vi "Rectangle Comparison.vi"(9 "Second":dbl[](array[numeric]), 11 "First":dbl[](array[numeric])) -> (0 "Rect":T1, 3 "Scores":T2)   [LabVIEW 2017]
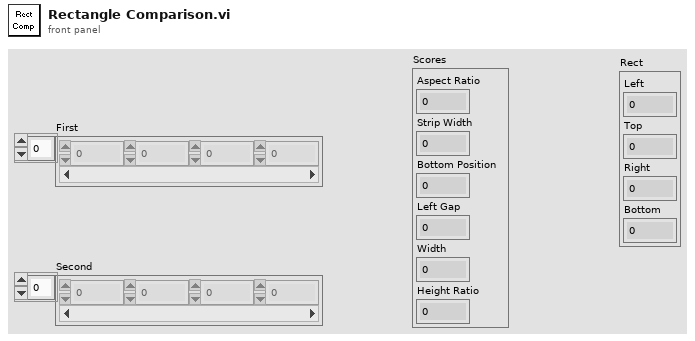
[diagram p1: front panel]
types:
  T1 = cluster{"Left":dbl, "Top":dbl, "Right":dbl, "Bottom":dbl}
  T2 = cluster{"Aspect Ratio":dbl, "Strip Width":dbl, "Bottom Position":dbl, "Left Gap":dbl, "Width":dbl, "Height Ratio":dbl}
  T3 = cluster{"[0]":dbl, "[1]":dbl, "[2]":dbl, "[3]":dbl}
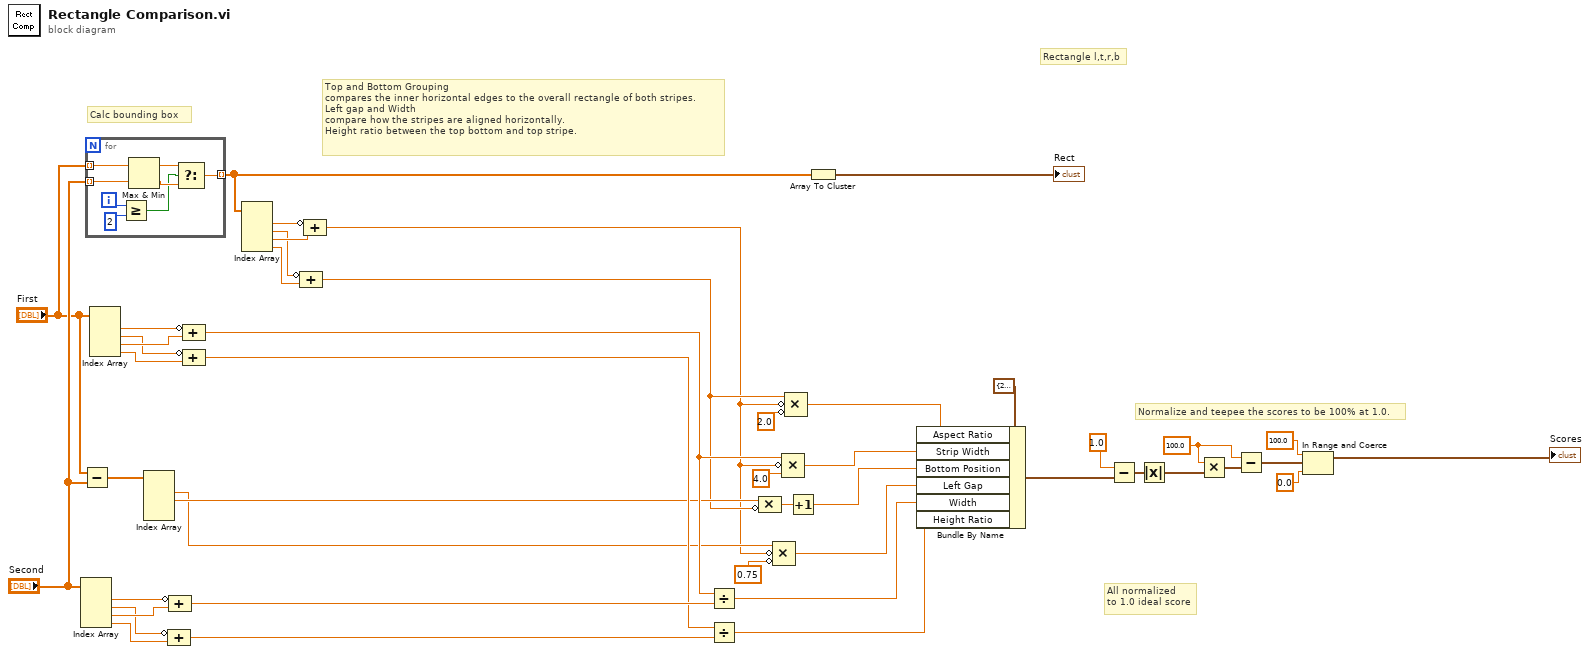
[diagram p0: block diagram]
diagram:
  w33 = 100.0 ("x/y")
  # "All normalized\nto 1.0 ideal score"
  # "Normalize and teepee the scores to be 100% at 1.0."
  # "Top and Bottom Grouping\ncompares the inner horizontal edges to the overall rectangle of both stripes.\nLeft gap and Width\ncompare how the stripes are aligned horizontally.\nHeight ratio between the top bottom and top stripe."
  # "Calc bounding box"
  # "Rectangle l,t,r,b"
  n1 = Index Array(array="Second") -> (element #1=w43:dbl, element #2=w24:dbl, element #3=w46:dbl, element #4=w8:dbl)  [unwired: 4 in]
  n2 = Subtract(x="First", y="Second") -> (x-y=w15:dbl[])
  n3 = for {
    tunnel: "First" -> [w54] mode=indexing
    tunnel: "Second" -> [w53] mode=indexing
    tunnel: [w47] -> w18 mode=indexing
    i -> [w51]
    n4 = Greater Or Equal?(x=w51, y=2) -> (x >= y?=w48:bool)
    n5 = Max & Min(x=w54, y=w53) -> (max(x,y)=w50:dbl, min(x,y)=w49:dbl)
    n6 = Select(t=w50, s=w48, f=w49) -> (s? t:f=w47:dbl)
  }
  n7 = Index Array(array="First") -> (element #1=w38:dbl, element #2=w23:dbl, element #3=w37:dbl, element #4=w39:dbl)  [unwired: 4 in]
  n8 = Index Array(array=w15) -> (element #1=w13:dbl, element #2=w14:dbl)  [unwired: 4 in, 2 out]
  n9 = Compound Arithmetic op=ADD(invert w24, w8) -> (w44:dbl)
  n10 = Compound Arithmetic op=ADD(invert w43, w46) -> (w45:dbl)
  n11 = Compound Arithmetic op=ADD(invert w38, w37) -> (w21:dbl)
  n12 = Compound Arithmetic op=ADD(invert w23, w39) -> (w25:dbl)
  n13 = Index Array(array=w18) -> (element #1=w10:dbl, element #2=w7:dbl, element #3=w9:dbl, element #4=w6:dbl)  [unwired: 4 in]
  n14 = Compound Arithmetic op=ADD(invert w7, w6) -> (w5:dbl)
  n15 = Compound Arithmetic op=ADD(invert w10, w9) -> (w4:dbl)
  n16 = Divide(x=w21, y=w45) -> (x/y=w41:dbl)
  n17 = Divide(x=w25, y=w44) -> (x/y=w40:dbl)
  n18 = Compound Arithmetic op=MULTIPLY(w14, invert w5) -> (w20:dbl)
  n19 = Compound Arithmetic op=MULTIPLY(w13, invert w4, invert 0.75 ("y")) -> (w16:dbl)
  n20 = Compound Arithmetic op=MULTIPLY(w21, invert w4, 4.0 ("y")) -> (w42:dbl)
  n21 = Compound Arithmetic op=MULTIPLY(w5, invert w4, invert 2.0 ("y")) -> (w1:dbl)
  n22 = Increment(x=w20) -> (x+1=w19:dbl)
  n23 = Array To Cluster(array=w18) -> (cluster=→"Rect":T3)
  n24 = Bundle By Name(cluster=T2 {"Aspect Ratio"=25.27472527472527, "Strip Width"=30.769230769230774, "Bottom Position"=34.78260869565217, "Left Gap"=76.92307692307692, "Width"=100.0, "Height Ratio"=68.75} ("Scores"), "Aspect Ratio"=w1, "Strip Width"=w42, "Bottom Position"=w19, "Left Gap"=w16, "Width"=w41, "Height Ratio"=w40) -> (w27:T2)
  n25 = Subtract(x=1.0 ("y"), y=w27) -> (x-y=w31:T2)
  n26 = Absolute Value(x=w31) -> (abs(x)=w34:T2)
  n27 = Multiply(x=w33, y=w34) -> (x*y=w35:T2)
  n28 = Subtract(x=w33, y=w35) -> (x-y=w30:T2)
  n29 = In Range and Coerce(upper limit=100.0, x=w30, lower limit=0.0) -> (coerced(x)=→"Scores":T2)  [unwired: 1 out]
